vi "FITS_ReadS32.vi"(8 "error in (no error)":errorcluster, 9 "Plane# (0..n-1)":u16, 10 "FITS":T2={"BITPIX"=8, "NAXIS"=2, "NAXIS1"=1, "NAXIS2"=1, "NAXIS3"=1, "BZERO"=0.0, "BSCALE"=1.0}, 11 "FITS file":T1) -> (0 "error out":errorcluster, 2 "Array":sgl[][](array[numeric]), 3 "Byte Stream File out":refnum<file>)   [LabVIEW 2011]
panel:
  out "x*y":dbl
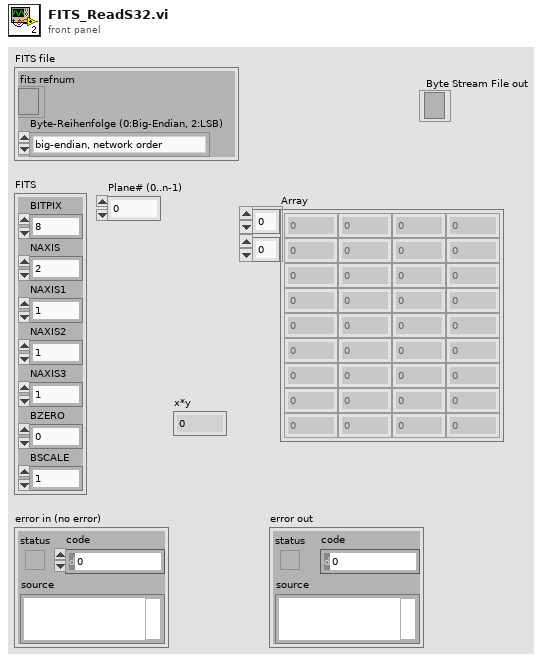
[diagram p1: front panel]
types:
  T1 = cluster{"fits refnum":refnum<file>, "Byte-Reihenfolge (0:Big-Endian, 2:LSB)":enum16{"big-endian, network order", "native, host order", "little-endian"}}
  T2 = cluster{"BITPIX":i16, "NAXIS":i16, "NAXIS1":u16, "NAXIS2":u16, "NAXIS3":u16, "BZERO":dbl, "BSCALE":dbl}
  T3 = enum16{"big-endian, network order", "native, host order", "little-endian"}
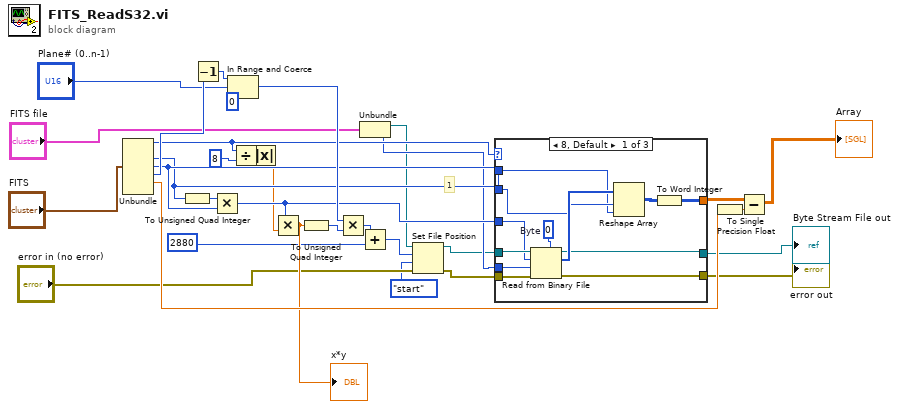
[diagram p0: block diagram]
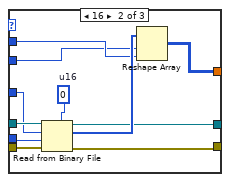
[diagram p2: hidden frame]
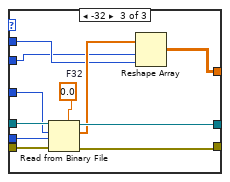
[diagram p3: hidden frame]
diagram:
  # "1"
  n1 = Unbundle("FITS") -> ("BITPIX"=w22:i16, "NAXIS1"=w13:u16, "NAXIS2"=w15:u16, "NAXIS3"=w26:u16, "BZERO"=w30:dbl)  [unwired: 2 out]
  n2 = To Unsigned Quad Integer(1:w13) -> (0:w23:u64)
  n3 = Decrement(x=w26) -> (x-1=w27:u16)
  n4 = Multiply(x=w23, y=w15) -> (x*y=w17:u64)
  n5 = In Range and Coerce(upper limit=w27, x="Plane# (0..n-1)", lower limit=u16 0) -> (coerced(x)=w24:u16)  [unwired: 1 out]
  n6 = Divide(x=w22, y=i16 8) -> (x/y=w16:dbl)
  n7 = Absolute Value(x=w16) -> (abs(x)=w1:dbl)
  n8 = Multiply(x=w17, y=w1) -> (x*y=w18:dbl)
  "x*y" <- w18
  n9 = To Unsigned Quad Integer(1:w18) -> (0:w20:u64)
  n10 = Multiply(x=w24, y=w20) -> (x*y=w19:u64)
  n11 = Unbundle("FITS file") -> ("fits refnum"=w6:refnum<file>, "Byte-Reihenfolge (0:Big-Endian, 2:LSB)"=w10:T3)
  n12 = Add(x=w19, y=2880) -> (x+y=w7:u64)
  n13 = Set File Position(offset (in bytes) (0)=w7, refnum=w6, from (0:start)=enum16{"start", "end", "current"}."start" ("pos mode (0:2)"), error in="error in (no error)") -> (refnum out=w9:refnum<file>, error out=w4:errorcluster)
  n14 = case shown="8, Default" w22 {
    tunnel: w13 -> [w33 w46 w57]
    tunnel: w15 -> [w34 w45 w56]
    tunnel: [w36 w55 w58] -> w29
    tunnel: w9 -> [w43 w54 w65]
    tunnel: w4 -> [w42 w53 w64]
    tunnel: [w41 w50 w61] -> w11
    tunnel: w17 -> [w38 w48 w62]
    tunnel: w10 -> [w37 w52 w63]
    tunnel: [w35 w47 w60] -> w12
    frame 8, Default {
      w39 = u8 0  # Byte
      n15 = Read from Binary File(5:w39, 8:w42, 9:w37, 10:w38, 11:w43) -> (0:w41:errorcluster, 2:w40:u8[], 3:w35:refnum<file>)  [unwired: 2 out]
      n16 = Reshape Array(w40, w34, w33) -> (w44:u8[][])
      n17 = To Word Integer(number=w44) -> (16bit integer=w36:i16[][])
    }
    frame 16 {
      w51 = u16 0  # u16
      n18 = Read from Binary File(5:w51, 8:w53, 9:w52, 10:w48, 11:w54) -> (0:w50:errorcluster, 2:w49:u16[], 3:w47:refnum<file>)  [unwired: 2 out]
      n19 = Reshape Array(w49, w45, w46) -> (w55:u16[][])
    }
    frame -32 {
      w66 = sgl 0.0  # F32
      n20 = Read from Binary File(5:w66, 8:w64, 9:w63, 10:w62, 11:w65) -> (0:w61:errorcluster, 2:w59:sgl[], 3:w60:refnum<file>)  [unwired: 2 out]
      n21 = Reshape Array(w59, w56, w57) -> (w58:sgl[][])
    }
  }
  "Byte Stream File out" <- w12
  "error out" <- w11
  n22 = To Single Precision Float(number=w30) -> (single precision float=w31:sgl)
  n23 = Subtract(x=w29, y=w31) -> (x-y=→"Array":sgl[][])
